vi "Get Routing Channel Initial State.vi"(8 "error in (no error)":errorcluster, 11 "Channel Ref in":T1 format="%.0x") -> (0 "error out":errorcluster, 2 "Initial State":string, 3 "Channel Ref out":T1=18446744073709551615 format="%.0x")   [LabVIEW 2017, in "Routing and Faulting Scripting.lvlib"]
uses:
  Routing and Faulting Scripting.lvlib
  <vilib>/NI Veristand/Custom Device API/Custom Device Item Ref.ctl
  <vilib>/Utility/error.llb/Error Cluster From Error Code.vi
  <vilib>/NI Veristand/Custom Device API/Custom Device API.lvlib
  Shared/Routing and Faulting Shared.lvlib
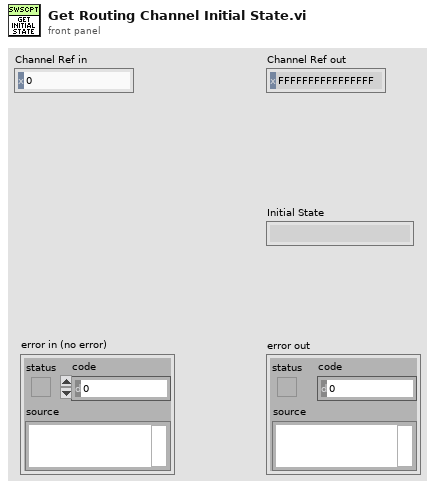
[diagram p1: front panel]
types:
  T1 = typedef "Custom Device API.lvlib/Custom Device Item Ref.ctl" = u64
  T2 = typedef "Custom Device API.lvlib/Custom Device Channel.ctl" = cluster{"Type":T3, "Units":string, "Default Value":dbl, "Faultable":bool, "Scalable":bool}
  T3 = typedef "Custom Device API.lvlib/Custom Device Channel Type.ctl" = enum16{"Input", "Output"}
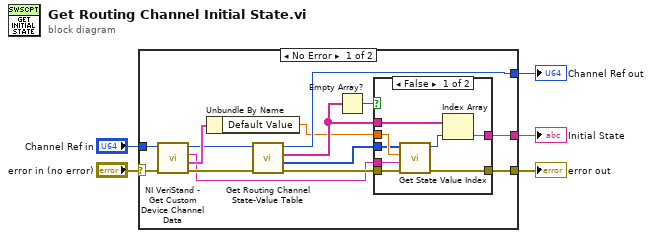
[diagram p0: block diagram]
diagram:
  n1 = case shown="No Error" "error in (no error)" {
    selector: "error in (no error)" -> [w17 w30]
    tunnel: [w11 w30] -> w2
    tunnel: "Channel Ref in" -> [w19 w29]
    tunnel: [w15 w29] -> w3
    tunnel: [w9 _] -> w1
    frame No Error {
      n2 = call <vilib>:"NI VeriStand - Get Custom Device Channel Data.vi"("error in (no error)"=w17, "Channel Ref in"=w19) -> ("error out"=w14:errorcluster, "Channel"=w18:T2, "Channel Name"=w8:string, "Channel Ref out"=w16:T1)  [unwired: 4 in, 2 out]
      n3 = Unbundle By Name(w18) -> ("Default Value"=w7:dbl)
      n4 = call "Get Routing Channel State-Value Table.vi"("error in (no error)"=w14, "Channel Ref in"=w16) -> ("error out"=w13:errorcluster, "State Values"=w6:i32[], "State Names"=w10:string[], "Channel Ref out"=w15:T1)  [unwired: 6 in]
      n5 = Empty Array?(array=w10) -> (empty?=w12:bool)
      n6 = case shown="False" w12 {
        tunnel: w13 -> [w27 w28]
        tunnel: w7 -> [w26 _]
        tunnel: w6 -> [w25 _]
        tunnel: [w24 w28] -> w11
        tunnel: w10 -> [w23 _]
        tunnel: [w21 _] -> w9
        tunnel: w8 -> [w20 _]
        frame False {
          n7 = call "Get State Value Index.vi"("error in (no error)"=w27, "Channel Name"=w20, "State Value"=w26, "State Value Array"=w25) -> ("error out"=w24:errorcluster, "index of element"=w22:i32)  [unwired: 6 in]
          n8 = Index Array(array=w23, index=w22) -> (element=w21:string)
        }
        frame True {
        }
      }
    }
    frame Error {
    }
  }
  "Channel Ref out" <- w3
  "error out" <- w2
  "Initial State" <- w1
